vi "do led runs.vi"() -> ()   [LabVIEW 2018]
panel:
  in  "Msg":string="WARNING: LABVIEW IS TAKING CONTROL OF PERIPHERALS\nTHE MOUSE WILL MOVE AND KEYSTROKES WILL BE SENT TO UPDATE THE LED INTENSITIES"
  out "Completed Runs":T1(array[cluster])
  out "Time to Next Run":string
  out "Elapsed Time In Current Run":string caption="Elapsed Time Text"
  out "error out":errorcluster
  in  "stop":bool
  in  "Queued Runs":T1(array[cluster])
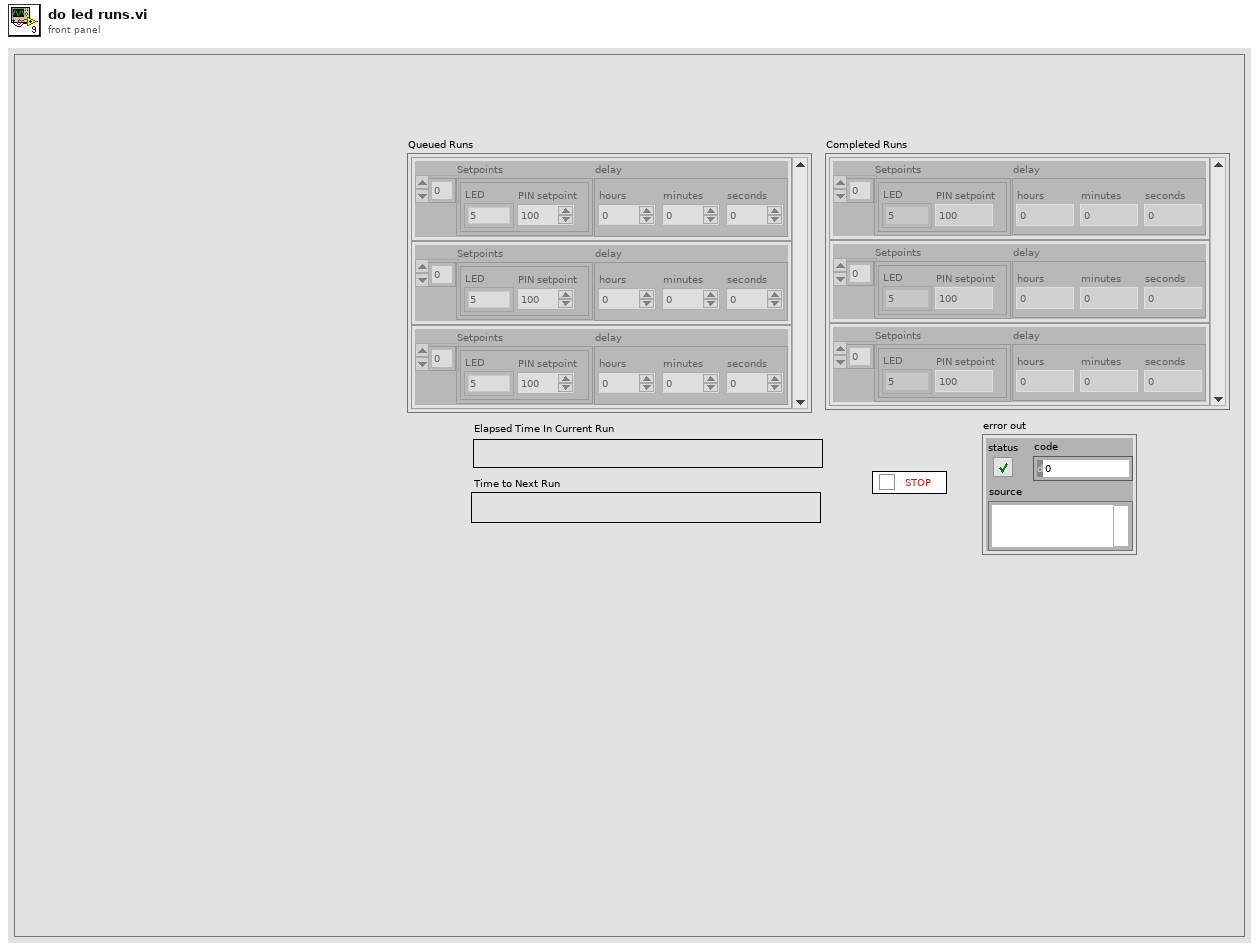
[diagram p1: front panel]
types:
  T1 = cluster{"Setpoints":cluster{"LED":enum16{"5", "6", "10", "13", "24", "28"}, "PIN setpoint":i32}[], "delay":cluster{"hours":i32, "minutes":i32, "seconds":i32}}[]
  T2 = cluster{"Setpoints":cluster{"LED":enum16{"5", "6", "10", "13", "24", "28"}, "PIN setpoint":i32}[], "delay":cluster{"hours":i32, "minutes":i32, "seconds":i32}}
  T3 = cluster{"LED":enum16{"5", "6", "10", "13", "24", "28"}, "PIN setpoint":i32}[]
  T4 = cluster{"hours":i32, "minutes":i32, "seconds":i32}
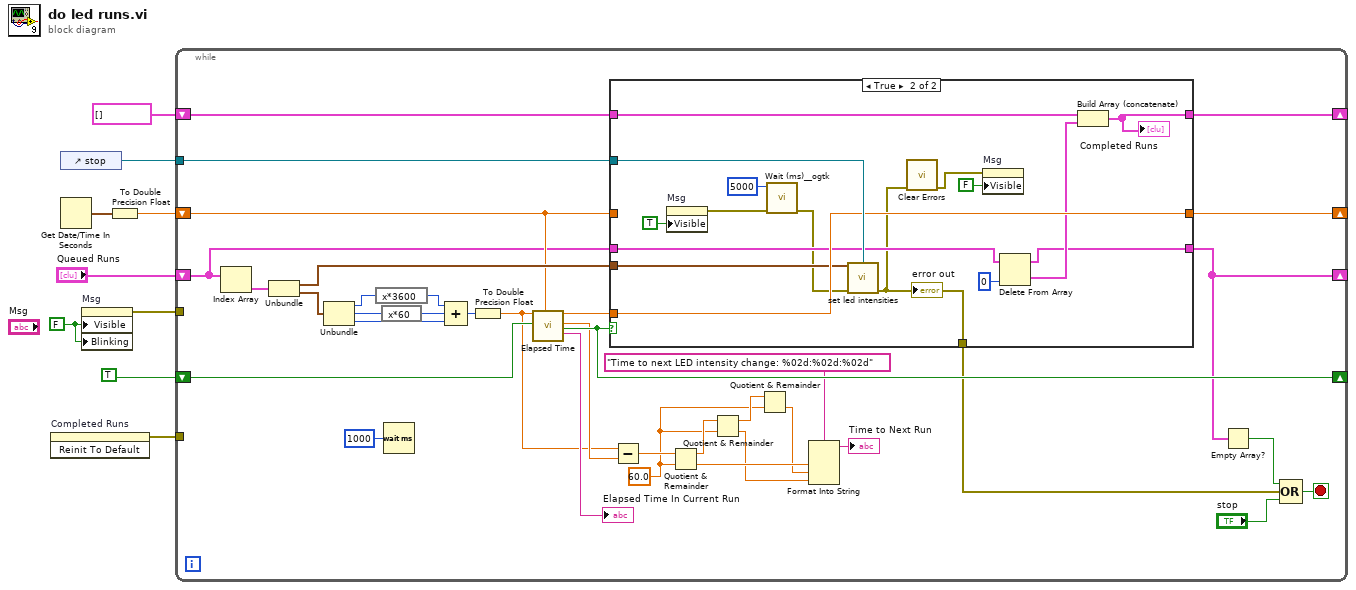
[diagram p0: block diagram]
diagram:
  w2 = FALSE ("Visible")
  n1 = invoke on="Completed Runs" class="Arr (strict)" method="Reinit To Default"() -> (error out=w3:errorcluster)  [unwired: 3 in, 2 out]
  n2 = control-ref of="stop"() -> (w5:refnum<vi>)
  n3 = Get Date/Time In Seconds() -> (seconds since 1Jan1904=w7:timestamp)
  n4 = property on="Msg" class="Str"("Visible"=w2, "Blinking"=w2) -> (error out=w1:errorcluster)  [unwired: 2 in, 1 out]
  n5 = To Double Precision Float(number=w7) -> (double precision float=w8:dbl)
  n6 = while {
    shift-right: [w11] -> _
    shift-left: "Queued Runs" -> [w15]
    shift-right: [w19] -> _
    shift-left: w8 -> [w17]
    shift-right: [w36] -> _
    shift-left: TRUE -> [w39]
    tunnel: w5 -> [w37]
    tunnel: w3 -> [_]
    shift-right: [w13] -> _
    shift-left: T1 [] ("Completed Runs") -> [w14]
    tunnel: w1 -> [_]
    stop <- w35 stop-if-true
    w25 = 60.0 ("y")
    n7 = Index Array(array=w15) -> (element=w16:T2)  [unwired: 1 in]
    n8 = Unbundle(w16) -> ("Setpoints"=w38:T3, "delay"=w45:T4)
    n9 = Unbundle(w45) -> ("hours"=w42:i32, "minutes"=w41:i32, "seconds"=w44:i32)
    n10 = expression code="x*3600"(w42) -> (w43:i32)
    n11 = expression code="x*60"(w41) -> (w40:i32)
    n12 = Wait (ms)(milliseconds to wait=u32 1000) -> ()  [unwired: 1 out]
    n13 = Compound Arithmetic op=ADD(w43, w40, w44) -> (w30:i32)
    n14 = To Double Precision Float(number=w30) -> (double precision float=w29:dbl)
    n15 = call "Elapsed Time"("Time Target (s)"=w29, "Reset"=w39, "Set Start Time (s)"=w17) -> ("Present (s)"=w18:dbl, "Elapsed Time (s)"=w31:dbl, "Time has Elapsed"=w36:bool, "Elapsed Time Text"=→"Elapsed Time In Current Run":string)  [unwired: 9 in, 4 out]
    n16 = case shown="True" w36 {
      tunnel: w38 -> [_ w57]
      tunnel: w37 -> [_ w64]
      tunnel: [_ w51] -> w34
      tunnel: [w48 w63] -> w19
      tunnel: w18 -> [_ w63]
      tunnel: w17 -> [w48 _]
      tunnel: w15 -> [w46 w62]
      tunnel: w14 -> [w47 w60]
      tunnel: [w47 w56] -> w13
      tunnel: [w46 w58] -> w11
      frame False {
      }
      frame True {
        n17 = property on="Msg" class="Str"("Visible"=TRUE) -> (error out=w54:errorcluster)  [unwired: 2 in, 1 out]
        n18 = call <userlib>:"Wait (ms)__ogtk.vi"("error in (no error)"=w54, "milliseconds to wait"=u32 5000) -> ("error out"=w53:errorcluster)  [unwired: 8 in, 1 out]
        n19 = call "set led intensities.vi"("Setpoints"=w57, "Abort Ref"=w64, "error in"=w53) -> ("error out"=w51:errorcluster)  [unwired: 12 in]
        "error out" <- w51
        n20 = call <vilib>:"Clear Errors.vi"("error in (no error)"=w51) -> ("error out"=w50:errorcluster)  [unwired: 5 in, 1 out]
        n21 = property on="Msg" class="Str"(error in=w50, "Visible"=FALSE) -> ()  [unwired: 1 in, 2 out]
        n22 = Delete From Array(array=w62, index=0) -> (deleted portion=w59:T2, array with subset deleted=w58:T1)  [unwired: 1 in]
        n23 = Build Array (concatenate)(w60, w59) -> (w56:T1)
        "Completed Runs" <- w56
      }
    }
    n24 = Subtract(x=w29, y=w31) -> (x-y=w28:dbl)
    n25 = Quotient & Remainder(x=w28, y=w25) -> (x-y*floor(x/y)=w27:dbl, floor(x/y)=w23:dbl)
    n26 = Quotient & Remainder(x=w27, y=w25) -> (x-y*floor(x/y)=w26:dbl, floor(x/y)=w21:dbl)
    n27 = Quotient & Remainder(x=w26, y=w25) -> (floor(x/y)=w22:dbl)  [unwired: 1 out]
    n28 = Format Into String(format string="Time to next LED intensity change: %02d:%02d:%02d", w23, w22, w21) -> (resulting string=→"Time to Next Run":string)  [unwired: 2 in, 1 out]
    n29 = Empty Array?(array=w11) -> (empty?=w10:bool)
    n30 = Compound Arithmetic op=OR(w10, w34, "stop") -> (w35:bool)
  }
